vi "Contents Summary Text.vi"(11 "Message":refnum<class "ErrorMessage.lvclass">) -> (2 "Contents Summary Text":string, 3 "Message":refnum<class "ErrorMessage.lvclass">)   [LabVIEW 2011, in "Messenging.lvlib" / "ErrorMessage.lvclass"]
uses:
  ErrorMessage.lvclass
  ErrorMessage.lvclass/ErrorMessage.ctl
  Parallel Process/Messsage Logger/Message Logger.lvclass
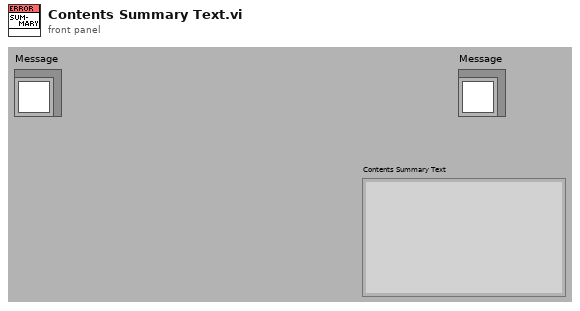
[diagram p1: front panel]
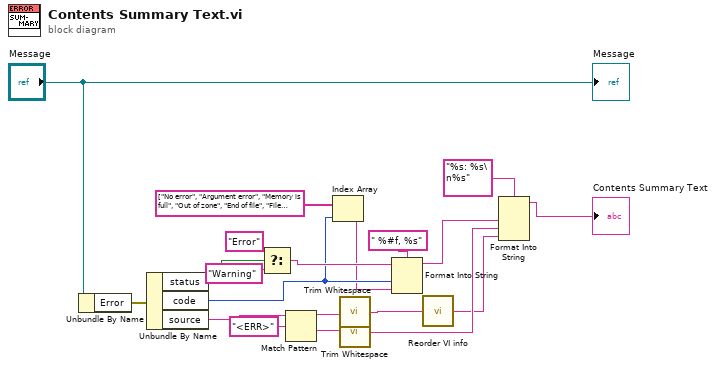
[diagram p0: block diagram]
diagram:
  n1 = Unbundle By Name("Message") -> ("Error"=w6:errorcluster)
  n2 = Unbundle By Name(w6) -> ("status"=w19:bool, "code"=w8:i32, "source"=w14:string)
  n3 = Select(t="Error", s=w19, f="Warning") -> (s? t:f=w15:string)
  n4 = Match Pattern(string=w14, regular expression="<ERR>") -> (before substring=w12:string, after substring=w11:string)  [unwired: 3 out]
  n5 = Index Array(array=string[] ["No error", "Argument error", "Memory is full", "Out of zone", "End of file", "File already open", "Generic file I/O error", "File not found", "File permission error", "Disk is full", "Duplicate path", "Too many files open", "System feature not enabled", "Resource file not found", "Cannot add resource", "Resource not found", "Image not found", "Image memory error", "Pen does not exist", "Config type invalid", "Config token not found", "Config parse error", "Config memory error", "Bad external code format", "Bad external code offset", "External code not present", "Null window", "Destroy window error", "Null menu", "Print aborted", "Bad print record", "Print driver error", "Windows error during printing", "Memory error during printing", "Print dialog error", "Generic print error", "Invalid device refnum", "Device not found", "Device parameter error", "Device unit error", "Cannot open device", "Device call aborted", "Generic error", "Cancelled by user", "Object ID too low", "Object ID too high", "Object not in heap", "Unknown heap", "Unknown object (invalid DefProc)", "Unknown object (DefProc not in table)", "Message out of range", "Invalid (null) method", "Unknown message", "Manager call not supported", "Bad address", "Network operation in progress", "Network operation timed out", "Connection is busy", "Network attribute not supported", "Network error", "Address in use", "System out of memory", "Connection aborted", "Connection refused", "Not connected", "Already connected", "Connection closed", "Initialization error (interapplication manager)", "Bad occurrence", "Wait on unbound occurrence handler", "Occurrence queue overflow", "Datalog type conflict", "Unused", "Unrecognized type (interapplication manager)", "Memory corrupt", "Failed to make temporary DLL", "Old CIN version", "Drag socket not found", "Failed to load drop-object", "Failed to register OLE object", "Failed to release OLE object", "Format specifier type mismatch", "Unknown format specifier", "Too few format specifiers", "Too many format specifiers", "Scan failed", "Newer CIN version", "Error converting to variant", "Runtime menu error", "Password tampered", "Variant attribute not found", "Incompatible variant data type", "Event data is not available", "Event Store is not present", "Occurrence is not found", "Event Queue is not created", "Event info is not available", "Refnum passed is NULL", "Error retrieving Class GUID", "Error retrieving CoClass GUID", "Error retrieving TypeLib GUID.", "Bad built application magic bytes.", "Specific driver is different from the specific driver associated with the Logical Name.", "There is no session opened to the class driver.", "Max Error", "MAX - Error with config objects", "MAX - Error loading configuration", "MAX - Group not supported"] ("Strings []"), index=w8) -> (element=w7:string)
  n6 = call <vilib>:"Trim Whitespace.vi"("string"=w12) -> ("trimmed string"=w10:string)  [unwired: 1 in]
  n7 = call <vilib>:"Trim Whitespace.vi"("string"=w11) -> ("trimmed string"=w3:string)  [unwired: 1 in]
  n8 = Format Into String(format string=" %#f, %s", initial string=w15, w8, w7) -> (resulting string=w4:string)  [unwired: 1 in, 1 out]
  n9 = call "Reorder VI info.vi"("chain"=w10) -> ("Reorderded"=w2:string)
  n10 = Format Into String(format string="%s: %s\n%s", w4, w3, w2) -> (resulting string=→"Contents Summary Text":string)  [unwired: 2 in, 1 out]
  "Message" <- "Message"
